vi "getBentStyle.vi"(0 "reference":refnum<class "ClassRelationshipEdge.lvclass">, 5 "error in (no error)":errorcluster) -> (14 "reference out":refnum<class "ClassRelationshipEdge.lvclass">, 15 "bentStyleRef":refnum<class "BentStyle.lvclass">, 19 "error out":errorcluster)   [LabVIEW 2014, in "ClassRelationshipEdge.lvclass"]
doc: "public BentStyle getBentStyle()"
uses:
  <resource>/Framework/Providers/Open_GDS/UML/ClassRelationshipEdge_class/ClassRelationshipEdge.lvclass
  <resource>/Framework/Providers/Open_GDS/UML/BentStyle_class/BentStyle.lvclass
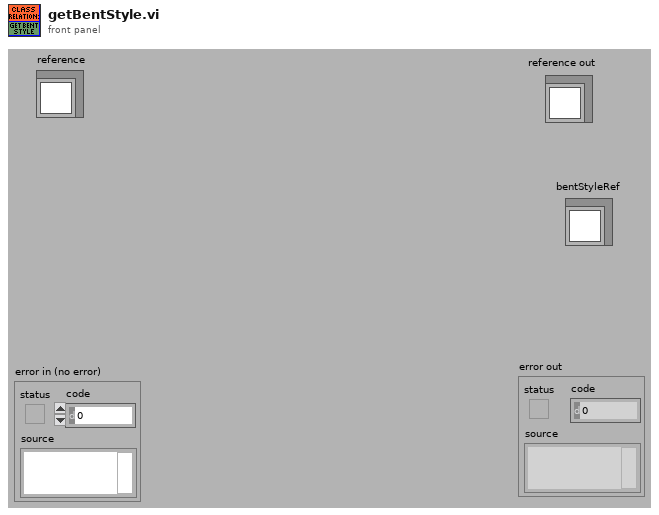
[diagram p1: front panel]
types:
  T1 = typedef "ClassRelationshipEdge.lvclass/ObjectAttributes.ctl" = cluster{"bentStyleRef":refnum<class "BentStyle.lvclass">, "startConnectionOffset":cluster{"x":i32, "y":i32}, "endConnectionOffset":cluster{"x":i32, "y":i32}, "MidLineOffset":cluster{"x":i32, "y":i32}, "DepClass":T2}
  T2 = typedef "ReversedEngineering_ViDependencyDetailsType.ctl" = cluster{"ThisVIs/Ctls":path[], "Dependent_VIs/Ctls":path[]}
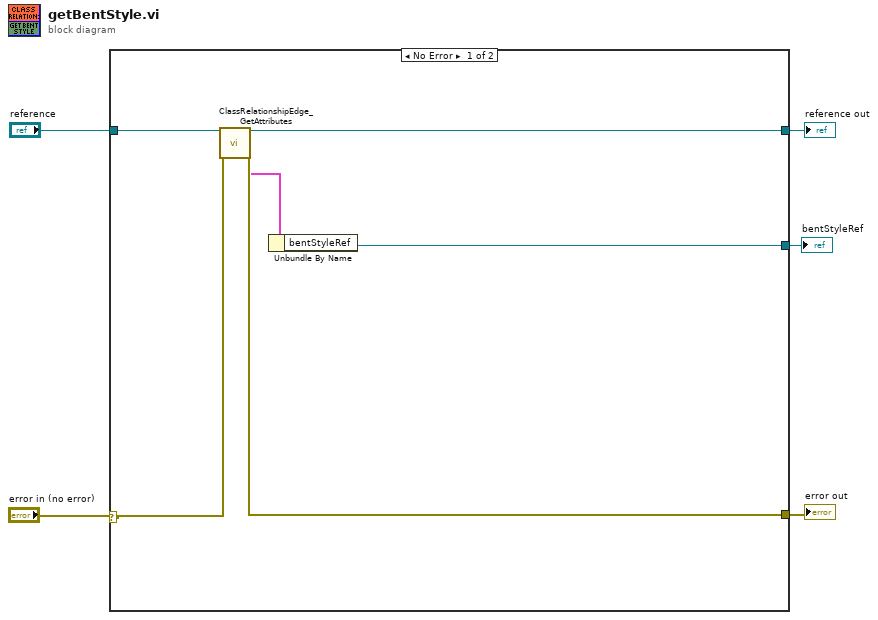
[diagram p0: block diagram]
diagram:
  n1 = case shown="No Error" "error in (no error)" {
    selector: "error in (no error)" -> [w7 w12]
    tunnel: "reference" -> [w11 w13]
    tunnel: [w10 w12] -> w4
    tunnel: [w9 w13] -> w3
    tunnel: [w8 _] -> w1
    frame No Error {
      n2 = call <resource>:"ClassRelationshipEdge_GetAttributes.vi"("reference in"=w11, "error in (no error)"=w7) -> ("reference out"=w9:refnum<class "ClassRelationshipEdge.lvclass">, "Data"=w6:T1, "error out"=w10:errorcluster)  [unwired: 1 in, 14 out]
      n3 = Unbundle By Name(w6) -> ("bentStyleRef"=w8:refnum<class "BentStyle.lvclass">)
    }
    frame Error {
    }
  }
  "reference out" <- w3
  "error out" <- w4
  "bentStyleRef" <- w1
